vi "svDataProcessing.vi"(6 "Z axis":dbl[](array[numeric]), 7 "Y axis":dbl[](array[numeric]), 8 "X axis":dbl[](array[numeric]), 9 "dt":dbl) -> (0 "PSD":cluster{"f0":dbl, "df":dbl, "magnitude":dbl[]}[](array[cluster]), 1 "statistical data":T1, 2 "Histogram Graph":T2(array[cluster]), 3 "Time data":waveform(dbl)[](array[waveform]))   [LabVIEW 2023]
uses:
  <vilib>/measure/maspectr.llb/Power Spectrum and PSD Export Mode.ctl
  <vilib>/Analysis/baseanly.llb/Mean (DBL).vi
  <vilib>/measure/maspectr.llb/FFT Power Spectrum and PSD for 1 Chan.vi
  <vilib>/Analysis/NI_AALBase.lvlib
  <vilib>/measure/NI_MAPro.lvlib
  <vilib>/gmath/NI_Gmath.lvlib
panel:
  out "Mean (all channels)":dbl[](array[numeric])
  out "Std (all channels)":dbl[](array[numeric])
  out "Variancce (all channels)":dbl[](array[numeric])
  out "Skewness (all channels)":dbl[](array[numeric])
  out "Kurtosis (all channels)":dbl[](array[numeric])
  out "Median Noise (all channels)":dbl[](array[numeric])
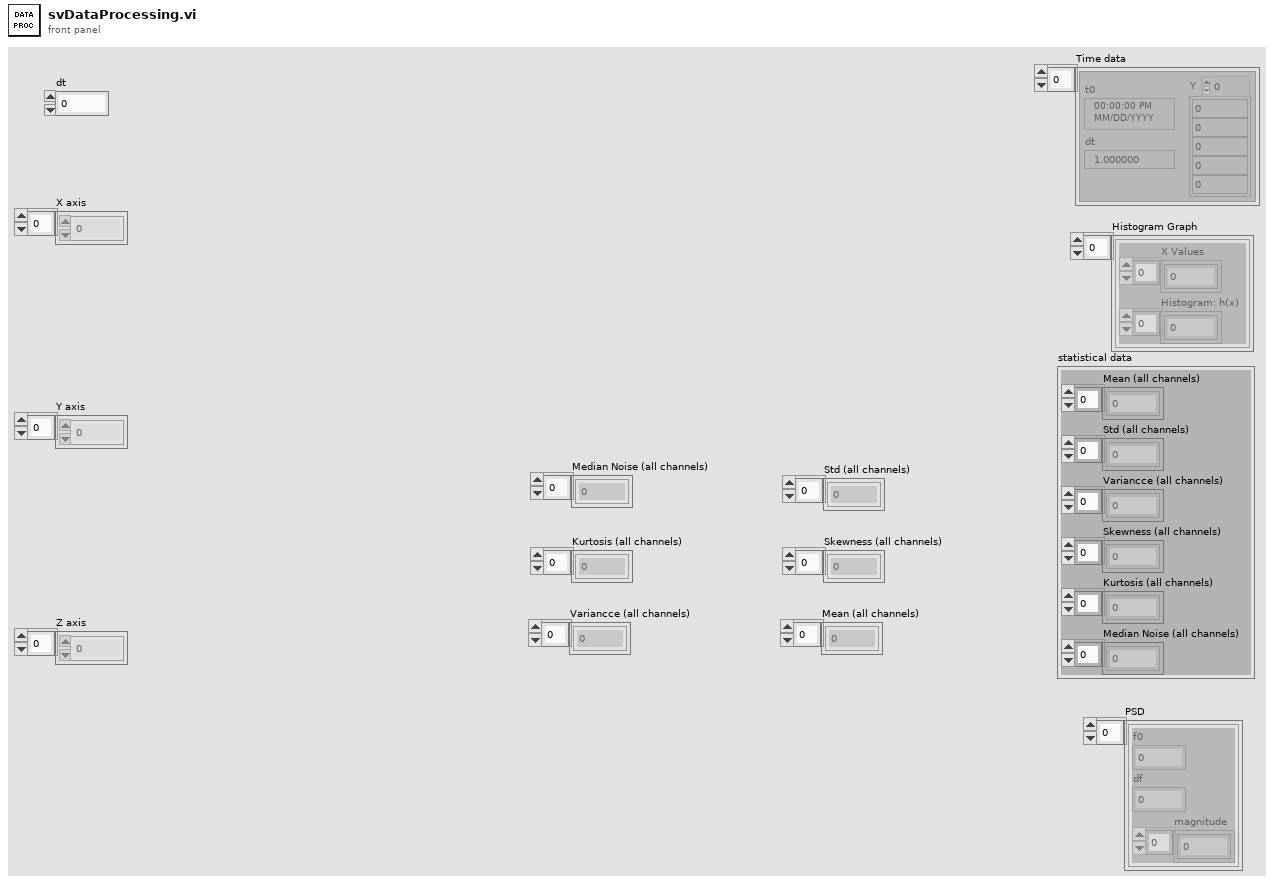
[diagram p1: front panel]
types:
  T1 = cluster{"Mean (all channels)":dbl[], "Std (all channels)":dbl[], "Variancce (all channels)":dbl[], "Skewness (all channels)":dbl[], "Kurtosis (all channels)":dbl[], "Median Noise (all channels)":dbl[]}
  T2 = cluster{"X Values":dbl[], "Histogram: h(x)":i32[]}[]
  T3 = typedef "NI_MAPro.lvlib/Power Spectrum and PSD Export Mode.ctl" = u16
  T4 = cluster{"X Values":dbl[], "Histogram: h(x)":i32[]}
  T5 = cluster{dbl[], dbl[], dbl[], dbl[], dbl[], dbl[]}
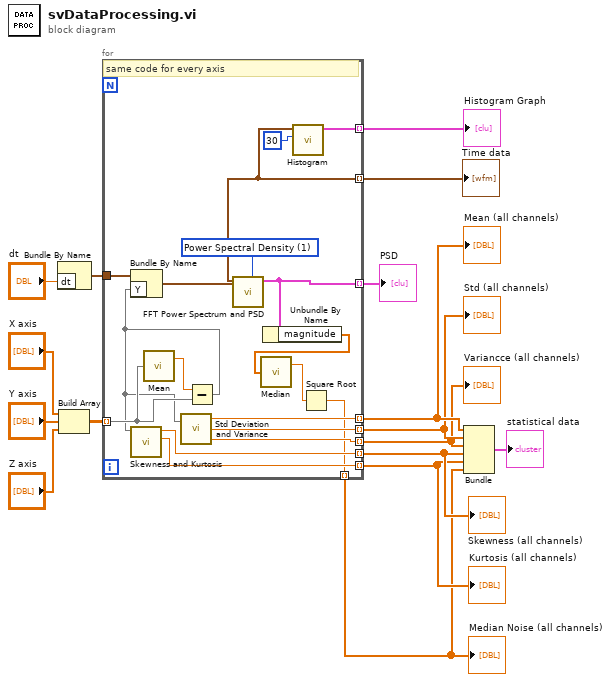
[diagram p0: block diagram]
diagram:
  n1 = Bundle By Name("dt"="dt") -> (w10:waveform(dbl))  [unwired: 1 in]
  n2 = Build Array("X axis", "Y axis", "Z axis") -> (w13:dbl[][])
  n3 = for {
    tunnel: w13 -> [w20] mode=indexing
    tunnel: w10 -> [w33]
    tunnel: [w30] -> w9 mode=indexing
    tunnel: [w31] -> w8 mode=indexing
    tunnel: [w23] -> w7 mode=indexing
    tunnel: [w24] -> w6 mode=indexing
    tunnel: [w29] -> w5 mode=indexing
    tunnel: [w28] -> w4 mode=indexing
    tunnel: [w26] -> w3 mode=indexing
    tunnel: [w25] -> w2 mode=indexing
    tunnel: [w17] -> w1 mode=indexing
    w27 = T3 1 items=["Power Spectrum", "Power Spectral Density"] ("export mode")
    # "same code for every axis"
    n4 = call-poly <vilib>:"Mean.vi"("X"=w20) -> ("mean"=w21:dbl)  [unwired: 1 out]
    n5 = Subtract(x=w21, y=w20) -> (x-y=w19:dbl[])
    n6 = Bundle By Name(cluster=w33, "Y"=w19) -> (w30:waveform(dbl))
    n7 = call <vilib>:"Skewness and Kurtosis.vi"("X"=w19) -> ("kurtosis"=w25:dbl, "skewness"=w26:dbl)  [unwired: 8 in, 1 out]
    n8 = call <vilib>:"Std Deviation and Variance.vi"("X"=w19) -> ("mean"=w24:dbl, "standard deviation"=w29:dbl, "variance"=w28:dbl)  [unwired: 1 in]
    n9 = call-poly <vilib>:"FFT Power Spectrum and PSD.vi"("export mode"=w27, "time signal"=w30) -> ("Power Spectrum / PSD"=w23:cluster{"f0":dbl, "df":dbl, "magnitude":dbl[]})  [unwired: 6 in, 3 out]
    n10 = Unbundle By Name(w23) -> ("magnitude"=w22:dbl[])
    n11 = call <vilib>:"Median.vi"("X"=w22) -> ("median"=w18:dbl)  [unwired: 1 out]
    n12 = call <vilib>:"Histogram.vi"("intervals"=30, "X"=w30) -> ("Histogram Graph"=w31:T4)  [unwired: 6 in, 3 out]
    n13 = Square Root(x=w18) -> (sqrt(x)=w17:dbl)
  }
  "Median Noise (all channels)" <- w1
  "PSD" <- w7
  "Kurtosis (all channels)" <- w2
  "Skewness (all channels)" <- w3
  "Variancce (all channels)" <- w4
  "Std (all channels)" <- w5
  "Mean (all channels)" <- w6
  "Histogram Graph" <- w8
  "Time data" <- w9
  n14 = Bundle(w6, w5, w4, w3, w2, w1) -> (→"statistical data":T5)  [unwired: 1 in]
